vi "check_file_exits.vi"(2 "error in (no error)":errorcluster, 3 "path":path) -> (0 "error out":errorcluster, 1 "file exists?":bool)   [LabVIEW 2018]
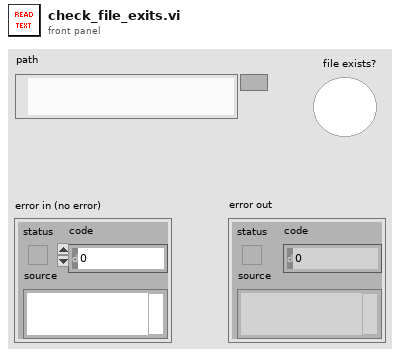
[diagram p1: front panel]
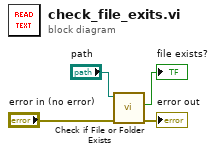
[diagram p0: block diagram]
diagram:
  n1 = call "Check if File or Folder Exists.vi"("error in (no error)"="error in (no error)", "path"="path") -> ("error out"=→"error out":errorcluster, "file or folder exists?"=→"file exists?":bool)  [unwired: 7 in, 1 out]
